vi "Validate_Destinations.vi"(8 "error in (no error)":errorcluster, 11 "AB_DepSourceDist in":refnum<class "AB_DepSourceDist.lvclass">) -> (0 "error out":errorcluster, 3 "AB_DepSourceDist out":refnum<class "AB_DepSourceDist.lvclass">)   [LabVIEW 2020, in "AB_DepSourceDist.lvclass"]
uses:
  <vilib>/AppBuilder/AB_Classes/DepSourceDist/AB_DepSourceDist.lvclass
  e:/builds/penguin/labview/branches/2020/dev/dist/vi.lib/AppBuilder/AB_Classes/Build/AB_Build.lvclass
  <vilib>/AppBuilder/AB_Classes/Build/AB_Build.lvclass
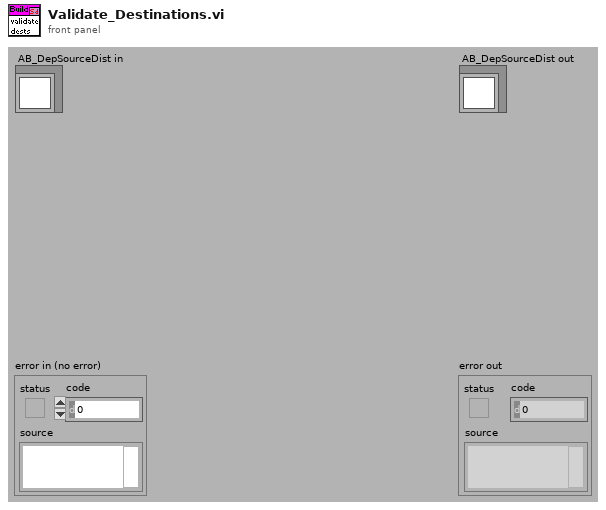
[diagram p1: front panel]
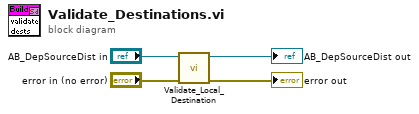
[diagram p0: block diagram]
diagram:
  n1 = call <vilib>:"Validate_Local_Destination.vi"("error in (no error)"="error in (no error)", "AB_Build in"="AB_DepSourceDist in") -> ("error out"=→"error out":errorcluster, "AB_Build out"=→"AB_DepSourceDist out":refnum<class "AB_DepSourceDist.lvclass">)  [unwired: 8 in]
